vi "SinWaveGen.vi"(8 "WaveTrough":dbl, 9 "WaveCrest":dbl=10.0, 10 "SinWavePeriod(Sec)":dbl=1.0, 11 "dt":dbl=0.01) -> (2 "SampleCount":i32, 3 "Waveform":waveform(dbl)(graph))   [LabVIEW 2024]
uses:
  <vilib>/Analysis/1siggen.llb/Ramp Pattern by Samples.vi
  <vilib>/gmath/NI_Gmath.lvlib
  <vilib>/Analysis/NI_AALBase.lvlib
panel:
  out "Waveform Graph 2":waveform(dbl)(graph)
  # "100 simples per sec"
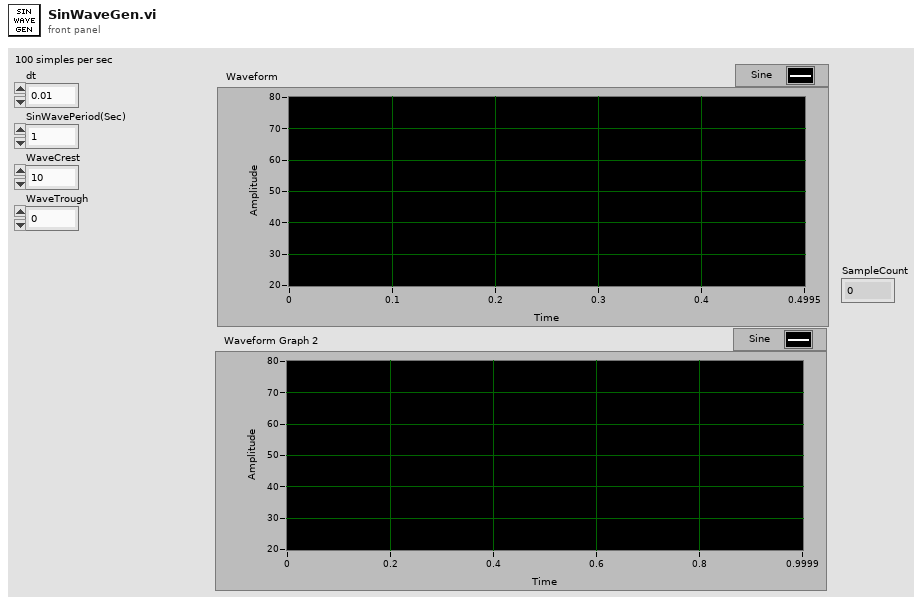
[diagram p1: front panel]
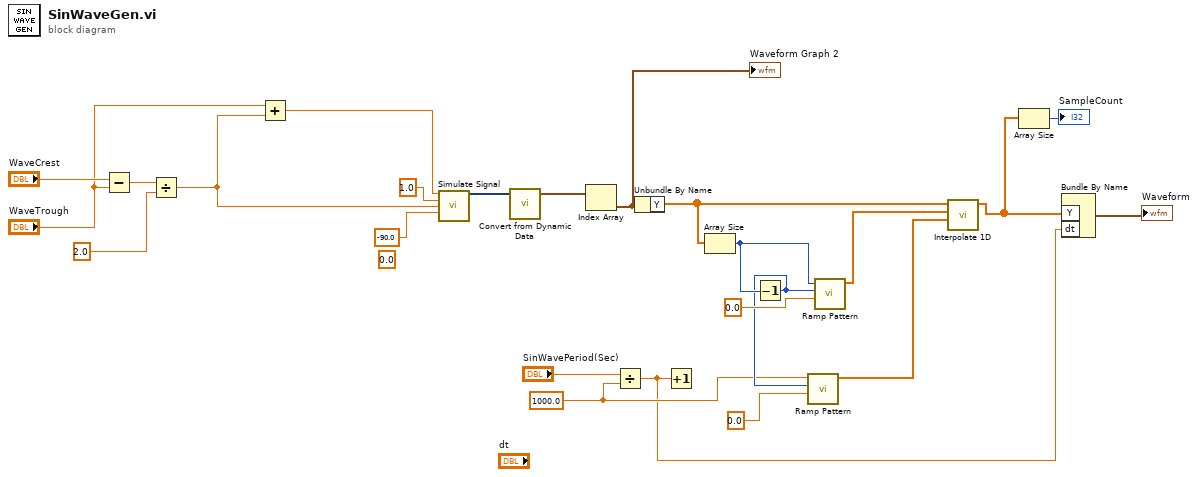
[diagram p0: block diagram]
diagram:
  w2 = 1000.0 ("x+1")
  (unwired) 0.0 ("Phase")
  n1 = Subtract(x="WaveCrest", y="WaveTrough") -> (x-y=w10:dbl)
  n2 = Divide(x=w10, y=2.0) -> (x/y=w6:dbl)
  n3 = Add(x="WaveTrough", y=w6) -> (x+y=w7:dbl)
  n4 = call "Simulate Signal"("Offset"=w7, "Frequency"=1.0, "Amplitude"=w6, "Phase"=-90.0) -> ("Sine"=w22:dynamicdata)  [unwired: 2 in, 9 out]
  n5 = call "Convert from Dynamic Data"("Dynamic Data Type"=w22) -> ("Array of Waveform"=w21:waveform(dbl)[])  [unwired: 3 out]
  n6 = Index Array(array=w21) -> (element=w14:waveform(dbl))  [unwired: 1 in]
  "Waveform Graph 2" <- w14
  n7 = Divide(x="SinWavePeriod(Sec)", y=w2) -> (x/y=w1:dbl)
  n8 = Unbundle By Name(w14) -> ("Y"=w19:dbl[])
  n9 = Increment(x=w1) -> ()  [unwired: 1 out]
  n10 = Array Size(array=w19) -> (size(s)=w4:i32)
  n11 = Decrement(x=w4) -> (x-1=w3:i32)
  n12 = call-poly <vilib>:"Ramp Pattern.vi"("start"=0.0, "end"=w3, "samples"=w2) -> ("Ramp Pattern"=w16:dbl[])  [unwired: 7 in, 1 out]
  n13 = call-poly <vilib>:"Ramp Pattern.vi"("start"=0.0, "end"=w3, "samples"=w4) -> ("Ramp Pattern"=w17:dbl[])  [unwired: 7 in, 1 out]
  n14 = call <vilib>:"Interpolate 1D.vi"("xi"=w16, "X"=w17, "Y"=w19) -> ("yi"=w13:dbl[])  [unwired: 6 in, 2 out]
  n15 = Array Size(array=w13) -> (size(s)=→"SampleCount":i32)
  n16 = Bundle By Name("Y"=w13, "dt"=w1) -> (→"Waveform":waveform(dbl))  [unwired: 1 in]
